vi "Open Subscription Policy.vi"(7 "Activate? (T)":bool=TRUE, 8 "error in (no error)":errorcluster, 10 "Transport":refnum<class "ITransport.lvclass">, 11 "SubscriptionPolicy":refnum<class "ISubscriptionPolicy.lvclass">) -> (0 "error out":errorcluster, 3 "Subscription Policy":T1)   [LabVIEW 2015, in "IMediator.lvlib" / "ISubscriptionPolicy.lvclass"]
doc: "<License>\nCopyright © 2017 Composed Systems, LLC | All rights reserved\nwww.composed.io\n\nAuthor: Ethan Stern <ethan.stern@composed.io>\n\nThis software is provided \"AS IS\" WITHOUT WARRANTIES, either express or implied, AND IS FOR EDUCATIONAL PURPOSES ONLY.\n</License>"
uses:
  ISubscriptionPolicy.lvclass
  ISubscriptionPolicy Reference.ctl
  ITransport/ITransport.lvclass
  ISubscriptionPolicy.lvclass/ISubscriptionPolicy.ctl
  <vilib>/Utility/error.llb/Error Cluster From Error Code.vi
  <vilib>/ErrorRing/Error Ring.xnode
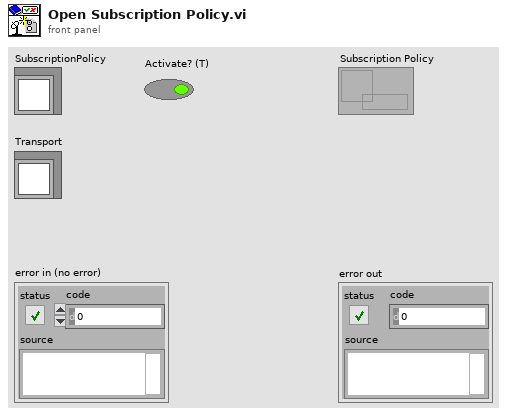
[diagram p1: front panel]
types:
  T1 = typedef "IMediator.lvlib/ISubscriptionPolicy.lvclass/ISubscriptionPolicy Reference.ctl" = refnum<data-value>
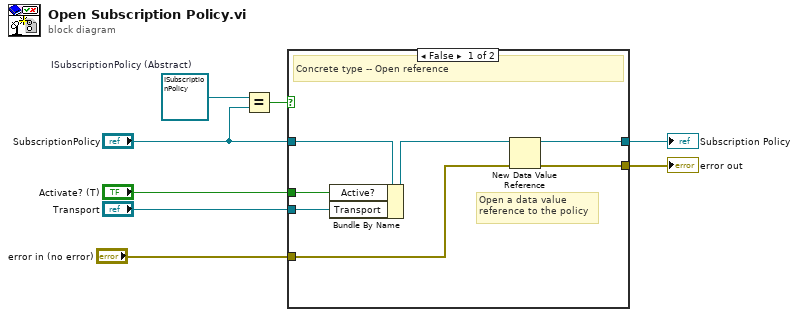
[diagram p0: block diagram]
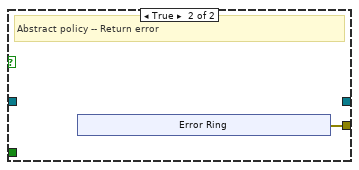
[diagram p2: hidden frame]
diagram:
  w4 = refnum<class "ISubscriptionPolicy.lvclass"> refnum  # ISubscriptionPolicy (Abstract)
  n1 = Equal?(x=w4, y="SubscriptionPolicy") -> (x = y?=w3:bool)
  n2 = case shown="False" w3 {
    tunnel: [w15 _] -> w8
    tunnel: [w14 w16] -> w7
    tunnel: "Transport" -> [w12 _]
    tunnel: "SubscriptionPolicy" -> [w11 _]
    tunnel: "Activate? (T)" -> [w10 _]
    tunnel: "error in (no error)" -> [w9 _]
    frame False {
      # "Open a data value\nreference to the policy"
      # "Concrete type -- Open reference"
      n3 = Bundle By Name(cluster=w11, "Active?"=w10, "Transport"=w12) -> (w13:refnum<class "ISubscriptionPolicy.lvclass">)
      n4 = New Data Value Reference(data value=w13, error in=w9) -> (data value reference=w15:refnum<data-value>, error out=w14:errorcluster)
    }
    frame True {
      # "Abstract policy -- Return error"
      n5 = xnode "Error Ring"() -> ("error out"=w16:errorcluster)
    }
  }
  "Subscription Policy" <- w8
  "error out" <- w7
